vi "CPP-5012Special.vi"() -> (5 "Plug in titles":string[](array[string]), 7 "Plug in values":string[](array[string]))   [LabVIEW 2011]
uses:
  Controls/Instrument_Array.ctl
  Globals/Meas_global.vi
  Globals/Plug_in_data_global.vi
  <vilib>/Utility/file.llb/Write To Spreadsheet File (DBL).vi
  <vilib>/Analysis/NI_AALBase.lvlib
panel:
  out "TimeTracePath":path
  in  "TimeTraceSaveLocation":path
  out "Compensated Stats":T1(array[cluster]) {"Min" format="%0.2f"; "Max" format="%0.2f"; "mean(5Maxs)" format="%0.2f"; "mean(5Mins)" format="%0.2f"; "SD(Cp)" format="%0.2f"; "meanCp" format="%0.2f"}
  out "Uncompensated Stats":T1(array[cluster]) {"Min" format="%0.2f"; "Max" format="%0.2f"; "mean(5Maxs)" format="%0.2f"; "mean(5Mins)" format="%0.2f"; "SD(Cp)" format="%0.2f"; "meanCp" format="%0.2f"}
  in  "ReferenceChannel":i32(ring)=3 items=["RV (t911)", "RV (t922)", "RV (t933)", "RV (t0)", "RV (t20)", "RV (t21)", "RV (t113)", "RV (t151)", "RV (t152)", "RV (t163)", "RV (t198)", "RV (t199)", "RV (t210)", "RV (t223)", "RV (t228)", "RV (t229)", "RV (t364)", "RV (t365)", "RV (t387)", "RV (t408)", "RV (t409)", "RV (t431)", "RV (t452)", "RV (t453)", "RV (t454)", "RV (t614)", "RV (t615)", "RV (t616)", "RV (t617)", "Save Nothing"]
  in  "ChsToCompensate":i32[](array[ring])=[0, 1, 2, 3, 4, 5, 6, 7, 8, 9, 10, 11, 12, 13, 14, 15, 16, 17, 18, 19, 20, 21, 22, 23, 23, 25, 26, 27, 28] items=["RV (t911)", "RV (t922)", "RV (t933)", "RV (t0)", "RV (t20)", "RV (t21)", "RV (t113)", "RV (t151)", "RV (t152)", "RV (t163)", "RV (t198)", "RV (t199)", "RV (t210)", "RV (t223)", "RV (t228)", "RV (t229)", "RV (t364)", "RV (t365)", "RV (t387)", "RV (t408)", "RV (t409)", "RV (t431)", "RV (t452)", "RV (t453)", "RV (t454)", "RV (t614)", "RV (t615)", "RV (t616)", "RV (t617)", "Off"]
  in  "ChannelZeroes":dbl[](array[numeric])=[2.2693, 2.3008, 2.3028, 2.2878, 2.3075, 2.3278, 2.2959, 2.3028, 2.2962, 2.2948, 2.2968, 2.3038, 2.2851, 2.2971, 2.2866, 2.2916, 2.3024, 2.3064, 2.2936, 2.2839, 2.3011, 2.2843, 2.3034, 2.2914, 2.2727, 2.2963, 2.3378, 2.2938, 2.3031]
  out "Mean(Pdyn)":dbl format="%0.2f"
  in  "Inst Array":T2=enum."Analogue"
  out "Graph":dbl[][](graph)
  out "ConcatenatingChannels:":i32[](array[ring])=[3] items=["RV (t911)", "RV (t922)", "RV (t933)", "RV (t0)", "RV (t20)", "RV (t21)", "RV (t113)", "RV (t151)", "RV (t152)", "RV (t163)", "RV (t198)", "RV (t199)", "RV (t210)", "RV (t223)", "RV (t228)", "RV (t229)", "RV (t364)", "RV (t365)", "RV (t387)", "RV (t408)", "RV (t409)", "RV (t431)", "RV (t452)", "RV (t453)", "RV (t454)", "RV (t614)", "RV (t615)", "RV (t616)", "RV (t617)", "Off"]
  # "Run this VI to update the channel names"
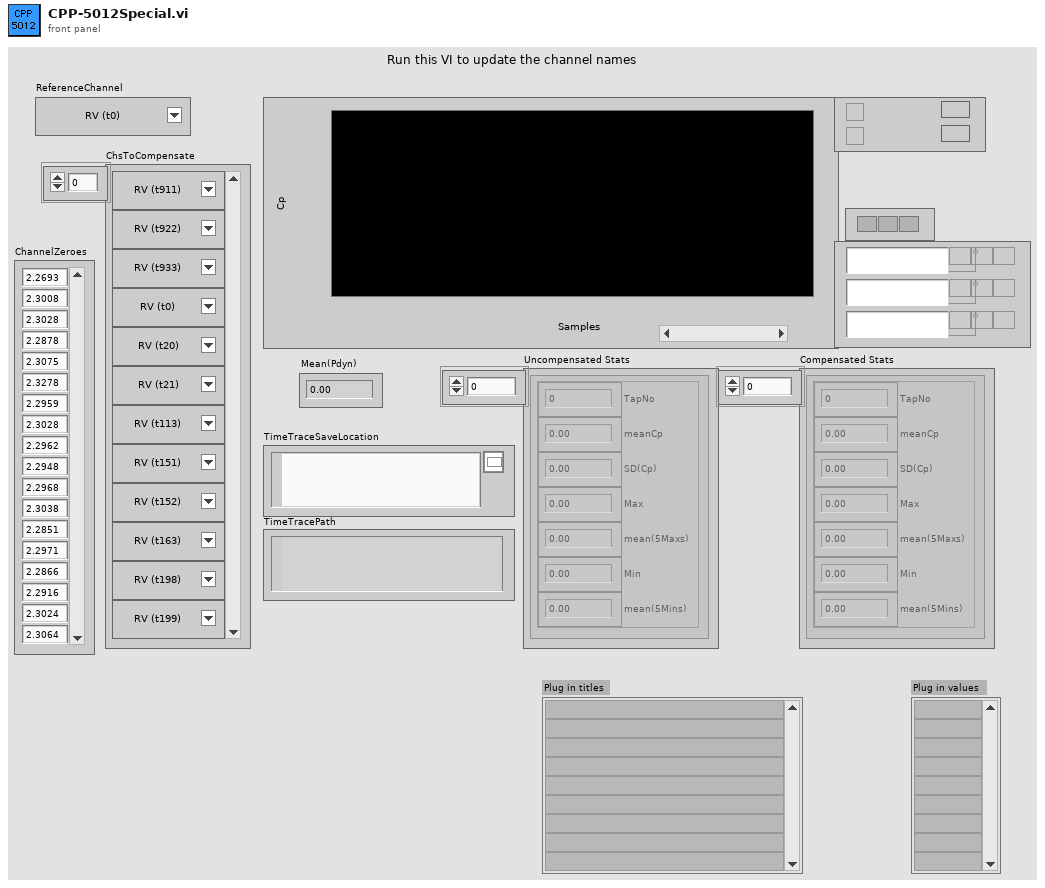
[diagram p1: front panel]
types:
  T1 = cluster{"TapNo":i32, "meanCp":dbl, "SD(Cp)":dbl, "Max":dbl, "mean(5Maxs)":dbl, "Min":dbl, "mean(5Mins)":dbl}[]
  T2 = typedef "Instrument_Array.ctl" = enum16{"PWA", "LDA", "Analogue"}
  T3 = typedef "Analysis_info_cluster.ctl" = cluster{"Colour":u32, "Inst type":T4, "Inst name":string, "Symbol":string, "Code name":string, "Extra Info":string, "Inst Array":T2, "Index":i32, "Voltage Index":i32, "Extra Titles":string[], "Extra Values":string[], "Eng Values":dbl[], "Time (ms)":dbl[], "TT / Voltage":dbl[], "U":dbl, "u^2":dbl, "u^3":dbl, "u^4":dbl, "Skew_u":dbl, "Kurt_u":dbl, "Mean % Err":dbl, "% u'/U":dbl}
  T4 = typedef "Inst_type.ctl" = enum16{"Propeller anemometer", "Raw voltage", "Pressure Transducer", "Pitot-static tube", "Preston tube", "Hot wire", "Cross wire 1", "Cross wire 2", "Generic Linear", "Generic Polynomial", "Generic BackPoly", "Fast FID", "Thermocouple", "Cold wire", "Pulsed Wire", "LDA Vel", "LDA Tran time", "LDA Arr time"}
  T5 = enum16{"Save no data", "Save data in new files", "Save data in existing files"}
  T6 = cluster{"TapNo":i32, "meanCp":dbl, "SD(Cp)":dbl, "Max":dbl, "mean(5Maxs)":dbl, "Min":dbl, "mean(5Mins)":dbl}
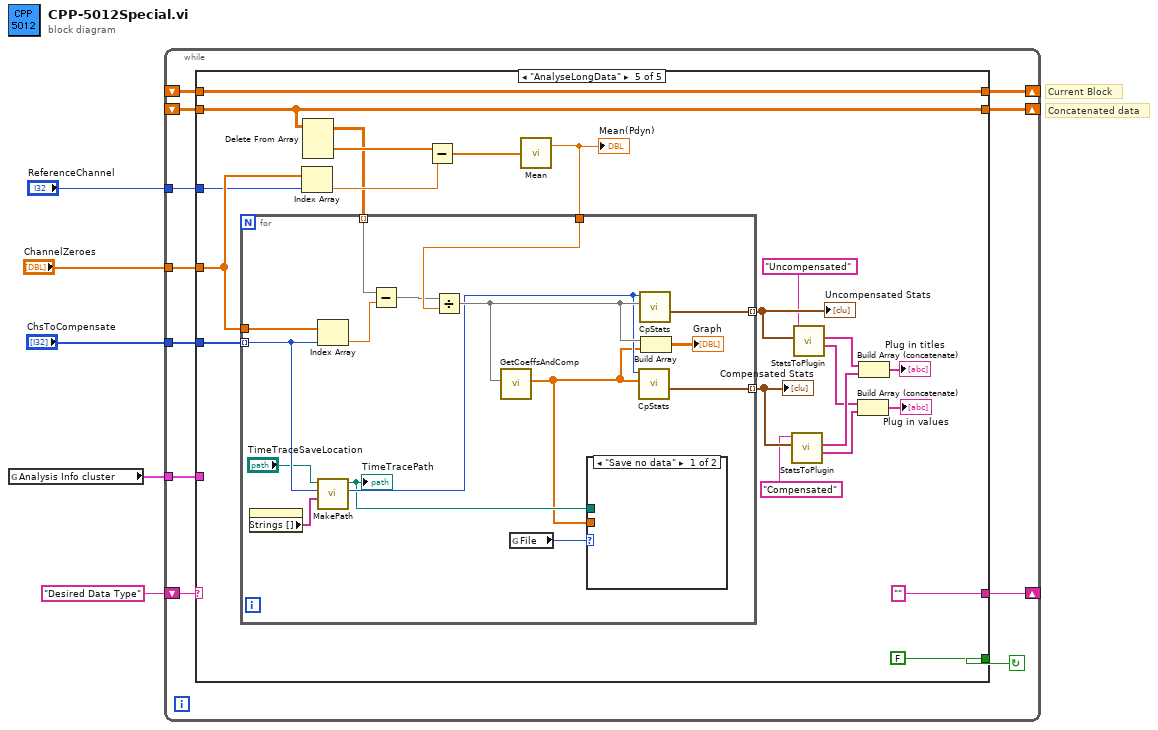
[diagram p0: block diagram]
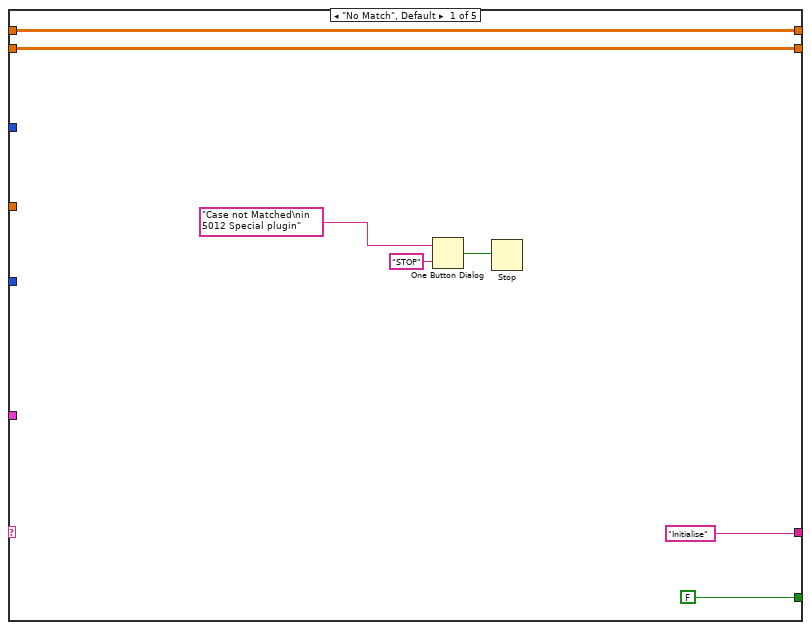
[diagram p2: hidden frame]
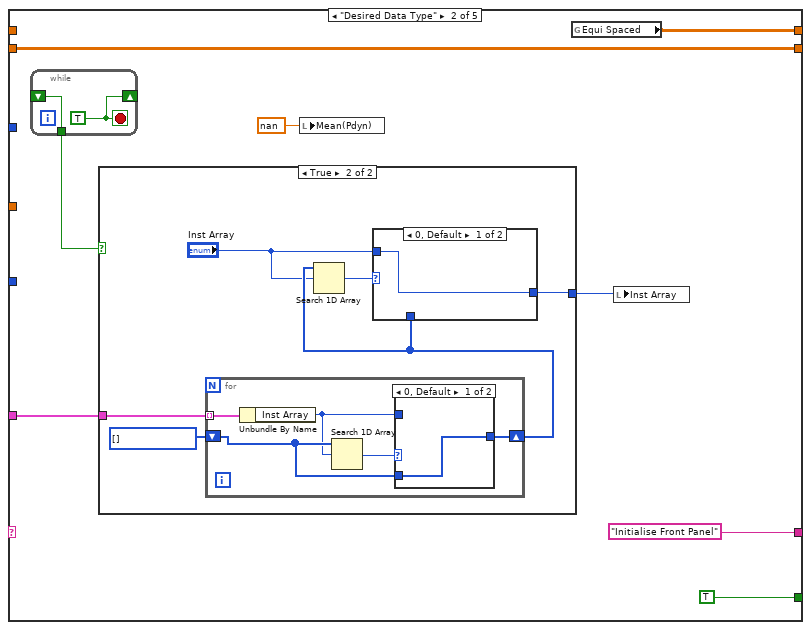
[diagram p3: hidden frame]
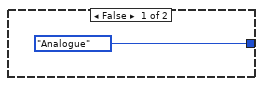
[diagram p4: hidden frame]
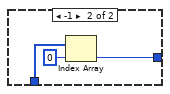
[diagram p5: hidden frame]
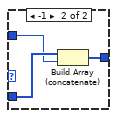
[diagram p6: hidden frame]
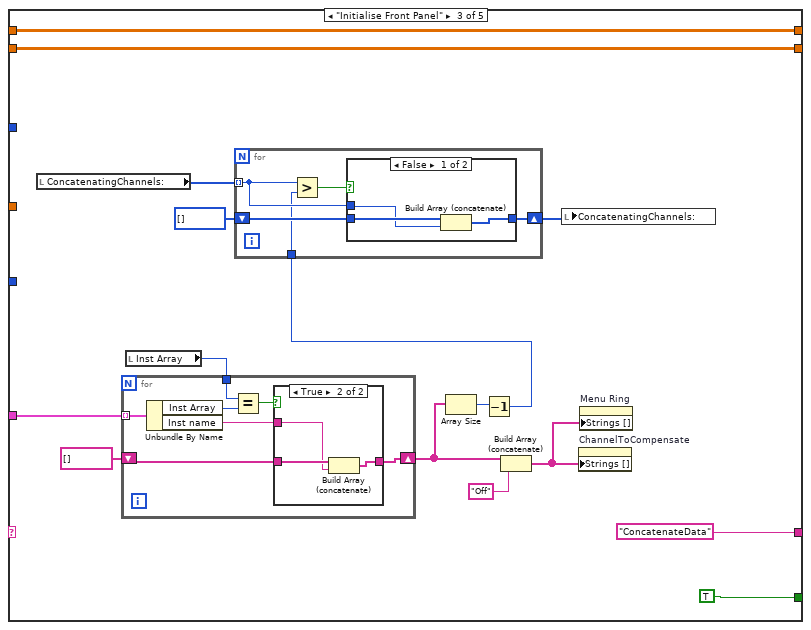
[diagram p7: hidden frame]
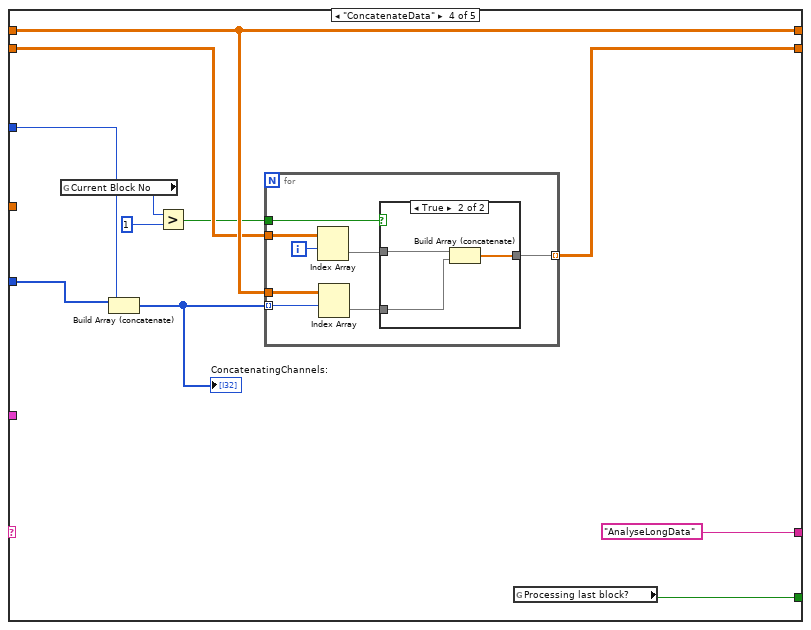
[diagram p10: hidden frame]
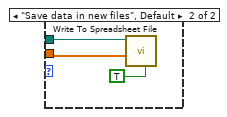
[diagram p12: hidden frame]
diagram:
  # "Concatenated data"
  # "Current Block"
  n1 = global read "Meas_global.vi" "Analysis Info cluster"() -> (w4:T3[])
  n2 = while {
    shift-left: "Desired Data Type" -> [w14]
    shift-right: [w15] -> _
    tunnel: w4 -> [w13]
    shift-right: [w12] -> _
    shift-left: _ -> [w11]
    shift-right: [w9] -> _
    shift-left: _ -> [w10]
    tunnel: "ReferenceChannel" -> [w8]
    tunnel: "ChsToCompensate" -> [w7]
    tunnel: "ChannelZeroes" -> [w6]
    stop <- w16 continue-if-true
    n3 = case shown="\"AnalyseLongData\"" w14 {
      tunnel: [FALSE TRUE TRUE w95 FALSE ("Processing last block?")] -> w16
      tunnel: ["Initialise" "Initialise Front Panel" "ConcatenateData" "AnalyseLongData" ("t") "" ("t")] -> w15
      tunnel: w13 -> [_ w27 w58 _ _]
      tunnel: [w19 w26 w62 w99 w133] -> w12
      tunnel: w11 -> [w19 _ w62 w99 w133]
      tunnel: w10 -> [w18 w29 w61 w98 w124]
      tunnel: [w18 w29 w61 w97 w124] -> w9
      tunnel: w8 -> [_ _ _ w89 w127]
      tunnel: w7 -> [_ _ _ w91 w129]
      tunnel: w6 -> [_ _ _ _ w128]
      frame "No Match", Default {
        n4 = One Button Dialog(message="Case not Matched\nin 5012 Special plugin" ("Format String"), button name ("OK")="STOP") -> (true=w21:bool)
        n5 = Stop(stop? (T)=w21) -> ()
      }
      frame "Desired Data Type" {
        n6 = while {
          shift-right: [w53] -> _
          shift-left: _ -> [w52]
          tunnel: [w52] -> w28
          stop <- w53 stop-if-true
          w53 = TRUE
        }
        n7 = case shown="True" w28 {
          tunnel: w27 -> [_ w38]
          tunnel: [Instrument_Array."Analogue" ("Inst Array") w34] -> w25
          frame False {
          }
          frame True {
            w37 = T2[] [] items=["PWA", "LDA", "Analogue"]
            n8 = for {
              tunnel: w38 -> [w47] mode=indexing
              shift-right: [w43] -> w35
              shift-left: w37 -> [w45]
              n9 = Unbundle By Name(w47) -> ("Inst Array"=w44:T2)
              n10 = Search 1D Array(1D array=w45, element=w44) -> (index of element=w46:i32)  [unwired: 1 out]
              n11 = case shown="0, Default" w46 {
                tunnel: w45 -> [w48 w51]
                tunnel: w44 -> [_ w50]
                tunnel: [w48 w49] -> w43
                frame 0, Default {
                }
                frame -1 {
                  n12 = Build Array (concatenate)(w51, w50) -> (w49:T2[])
                }
              }
            }
            n13 = Search 1D Array(1D array=w35, element="Inst Array") -> (index of element=w36:i32)  [unwired: 1 out]
            n14 = case shown="0, Default" w36 {
              tunnel: w35 -> [_ w41]
              tunnel: [w39 w40] -> w34
              tunnel: "Inst Array" -> [w39 _]
              frame 0, Default {
              }
              frame -1 {
                n15 = Index Array(array=w41, index=0) -> (element=w40:T2)
              }
            }
          }
        }
        n16 = local write "Mean(Pdyn)"(nan ("Channel'sZero")) -> ()
        n17 = global read "Plug_in_data_global.vi" "Equi Spaced"() -> (w26:dbl[][])
        n18 = local write "Inst Array"(w25) -> ()
      }
      frame "Initialise Front Panel" {
        n19 = local read "ConcatenatingChannels:"() -> (w68:i32[])
        n20 = local read "Inst Array"() -> (w57:T2)
        n21 = for {
          tunnel: w57 -> [w74]
          tunnel: w58 -> [w73] mode=indexing
          shift-right: [w70] -> w56
          shift-left: string[] [] -> [w71]
          n22 = Unbundle By Name(w73) -> ("Inst Array"=w75:T2, "Inst name"=w69:string)
          n23 = Equal?(x=w74, y=w75) -> (x = y?=w72:bool)
          n24 = case shown="True" w72 {
            tunnel: w71 -> [w76 w79]
            tunnel: [w76 w78] -> w70
            tunnel: w69 -> [_ w77]
            frame False {
            }
            frame True {
              n25 = Build Array (concatenate)(w79, w77) -> (w78:string[])
            }
          }
        }
        n26 = Array Size(array=w56) -> (size(s)=w64:i32)
        n27 = Decrement(x=w64) -> (x-1=w63:i32)
        n28 = for {
          tunnel: w68 -> [w81] mode=indexing
          shift-right: [w82] -> w66
          shift-left: i32[] [] -> [w83]
          tunnel: w63 -> [w80]
          n29 = Greater?(x=w81, y=w80) -> (0:w84:bool)
          n30 = case shown="False" w84 {
            tunnel: w83 -> [w87 w88]
            tunnel: [w86 w88] -> w82
            tunnel: w81 -> [w85 _]
            frame False {
              n31 = Build Array (concatenate)(w87, w85) -> (w86:i32[])
            }
            frame True {
            }
          }
        }
        n32 = Build Array (concatenate)(w56, "Off") -> (w54:string[])
        n33 = local write "ConcatenatingChannels:"(w66) -> ()
        n34 = property on="ChannelToCompensate" class="Ring (strict)"("Strings []"=w54) -> ()  [unwired: 2 in, 2 out]
        n35 = property on="Menu Ring" class="Ring (strict)"("Strings []"=w54) -> ()  [unwired: 2 in, 2 out]
      }
      frame "ConcatenateData" {
        n36 = global read "Meas_global.vi" "Current Block No"() -> (w94:i32)
        n37 = Build Array (concatenate)(w91, w89) -> (w90:i32[])
        "ConcatenatingChannels:" <- w90
        n38 = Greater?(x=w94, y=1) -> (0:w92:bool)
        n39 = for {
          tunnel: w99 -> [w107]
          tunnel: w90 -> [w106] mode=indexing
          tunnel: w98 -> [w103]
          tunnel: [w104] -> w97 mode=indexing
          tunnel: w92 -> [w105]
          i -> [w102]
          n40 = Index Array(array=w103, index (row)=w102) -> (element=w101:dbl[])  [unwired: 1 in]
          n41 = Index Array(array=w107, index (row)=w106) -> (element=w100:dbl[])  [unwired: 1 in]
          n42 = case shown="True" w105 {
            tunnel: w101 -> [_ w111]
            tunnel: w100 -> [w108 w110]
            tunnel: [w108 w109] -> w104
            frame False {
            }
            frame True {
              n43 = Build Array (concatenate)(w111, w110) -> (w109:dbl[])
            }
          }
        }
        n44 = global read "Meas_global.vi" "Processing last block?"() -> (w95:bool)
      }
      frame "AnalyseLongData" {
        n45 = Index Array(array=w128, index=w127) -> (element=w126:dbl)
        n46 = Delete From Array(array=w124) -> (deleted portion=w125:dbl[], array with subset deleted=w123:dbl[][])  [unwired: 3 in]
        n47 = Subtract(x=w125, y=w126) -> (x-y=w122:dbl[])
        n48 = call <vilib>:"Mean.vi"("X"=w122) -> ("mean"=w130:dbl)  [unwired: 1 out]
        "Mean(Pdyn)" <- w130
        n49 = for {
          tunnel: w130 -> [w148]
          tunnel: w129 -> [w141] mode=indexing
          tunnel: w123 -> [w144] mode=indexing
          tunnel: w128 -> [w145]
          tunnel: [w139] -> w121 mode=indexing
          tunnel: [w138] -> w119 mode=indexing
          n50 = property on="ChannelToCompensate" class="Ring (strict)"() -> ("Strings []"=w142:string[])  [unwired: 2 in, 2 out]
          n51 = Index Array(array=w145, index=w141) -> (element=w149:dbl)
          n52 = call "MakePath.vi"("Strings []"=w142, "ChannelToCompensate"=w141, "TimeTraceSaveLocation"="TimeTraceSaveLocation") -> ("RV number"=w140:i32, "appended path"=w136:path)  [unwired: 7 in]
          "TimeTracePath" <- w136
          n53 = Subtract(x=w144, y=w149) -> (x-y=w147:dbl[])
          n54 = Divide(x=w147, y=w148) -> (x/y=w143:dbl[])
          n55 = call "GetCoeffsAndComp.vi"("mutedData"=w143) -> ("boostedData"=w135:dbl[])  [unwired: 10 in]
          n56 = global read "Meas_global.vi" "File"() -> (w134:T5)
          n57 = case shown="\"Save no data\"" w134 {
            tunnel: w136 -> [_ w152]
            tunnel: w135 -> [_ w151]
            frame "Save no data" {
            }
            frame "Save data in new files", Default {
              n58 = call-poly <vilib>:"Write To Spreadsheet File.vi"("transpose? (no:F)"=TRUE, "1D data"=w151, "file path (dialog if empty)"=w152) -> ()  [unwired: 5 in, 1 out]
            }
          }
          n59 = call "CpStats.vi"("Cp=P/Pdyn"=w135, "TapNo"=w140) -> ("StatsCluster"=w138:T6)  [unwired: 9 in]
          n60 = call "CpStats.vi"("Cp=P/Pdyn"=w143, "TapNo"=w140) -> ("StatsCluster"=w139:T6)  [unwired: 9 in]
          n61 = Build Array(w143, w135) -> (→"Graph":dbl[][])
        }
        "Uncompensated Stats" <- w121
        "Compensated Stats" <- w119
        n62 = call "StatsToPlugin.vi"("Stats"=w119, "AdditionalNote"="Compensated") -> ("Plug in values"=w115:string[], "Plug in titles"=w116:string[])  [unwired: 8 in]
        n63 = call "StatsToPlugin.vi"("Stats"=w121, "AdditionalNote"="Uncompensated") -> ("Plug in values"=w114:string[], "Plug in titles"=w117:string[])  [unwired: 8 in]
        n64 = Build Array (concatenate)(w114, w115) -> (→"Plug in values":string[])
        n65 = Build Array (concatenate)(w117, w116) -> (→"Plug in titles":string[])
      }
    }
  }
